vi "20210716_Scan with scanning mirror_center point_ver4.0.vi"(8 "Y Scan range (V)":dbl=0.2 min=-200.0 max=300.0, 9 "X Scan range (V)":dbl=0.2 min=-200.0 max=300.0, 10 "Y center (V)":dbl min=-200.0 max=300.0, 11 "X center (V)":dbl min=-200.0 max=300.0) -> ()   [LabVIEW 2015]
uses:
  Libraries/SR400/Public/Typedefs/Counter.ctl
  <vilib>/Analysis/1siggen.llb/Ramp Pattern by Samples.vi
  <vilib>/Analysis/NI_AALBase.lvlib
  Libraries/SR400/SR400.lvlib
panel:
  in  "file path":path
  out "SR400 counts":dbl
  in  "STOP\nSCAN":bool
  in  "Position from":enum16{"Left", "Right", "Control"}(ring)
  in  "Scan select":enum16{"Left", "Right"}(ring)
  in  "Position select":enum16{"Left", "Right", "Zero", "Control"}(ring)
  out "Current Y position (V)":dbl format="%#_4g"
  out "Current X position (V)":dbl format="%#_4g"
  out "Cursor_Y (V) 2":dbl format="%#.5f"
  out "Cursor_X (V) 2":dbl format="%#.5f"
  out "Cursor_Y position 2":i32
  out "Cursor_X position 2":i32
  out "X_Array 2":dbl[](array[numeric])
  out "Y_Array 2":dbl[](array[numeric])
  out "Rescanned Intensity Graph":dbl[][](graph)
  out "Count plot":dbl(graph)=137.0
  in  "stop monitoring":bool
  in  "Log":bool
  out "X_Array":dbl[](array[numeric])
  out "Y_Array":dbl[](array[numeric])
  in  "Scan":bool
  out "Cursor_Y (V)":dbl format="%#.5f"
  out "Cursor_X (V)":dbl format="%#.5f"
  in  "Go":bool
  in  "Stop program":bool
  out "Cursor_Y position":i32
  out "Cursor_X position":i32
  in  "Count Time Set":dbl[unit]=0.01
  in  "# of average":i32=1
  in  "VISA resource name":refnum<visa-resource-name>="GPIB0::18::INSTR"
  in  "Dwell time (ms)":i32=2
  out "Counts":dbl
  in  "Time delay bet. movement\n& measurement (ms)":i32=1
  in  "X data number(Ao1)":i32=150
  out "Max Value":dbl format="%#.2p"
  out "Max Y (V)":dbl format="%#.5f"
  out "Max X (V)":dbl format="%#.5f"
  out "Intensity Graph":dbl[][](graph)
  out "ao1_V":dbl
  out "ao1_index":i32
  out "ao0_V":dbl
  out "ao0_index":i32
  in  "Y data number(Ao0)":i32=150
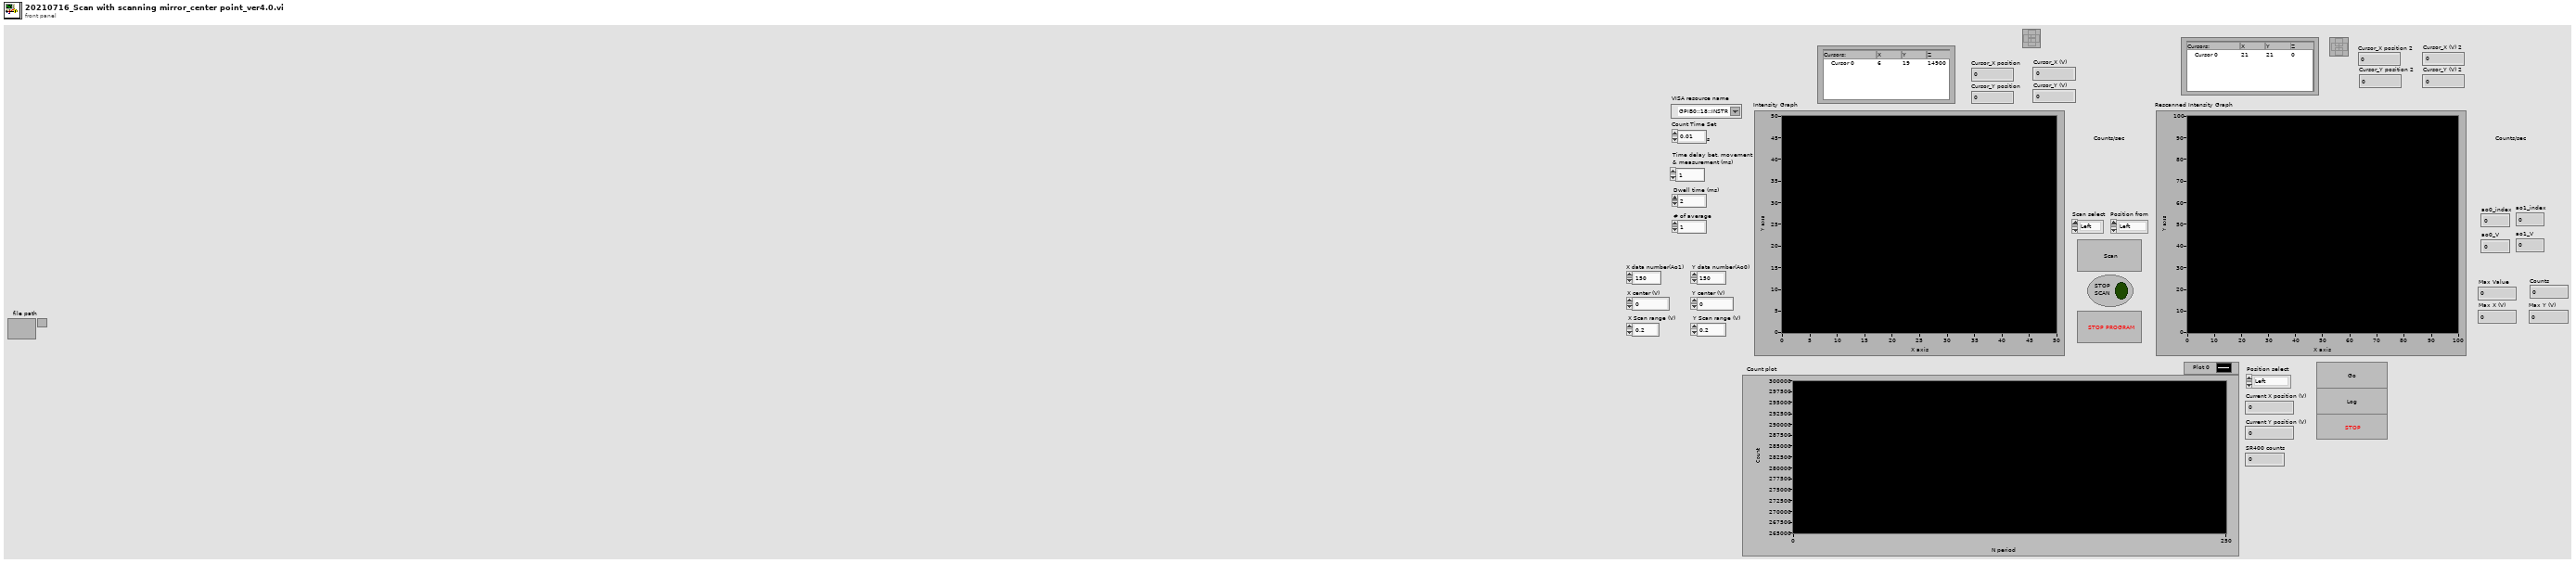
[diagram p1: front panel]
types:
  T1 = enum16{"open", "open or create", "create or replace", "create", "open (read only)"}
  T2 = typedef "SR400.lvlib/Counter.ctl" = enum16{"Counter A", "Counter B", "Counter T"}
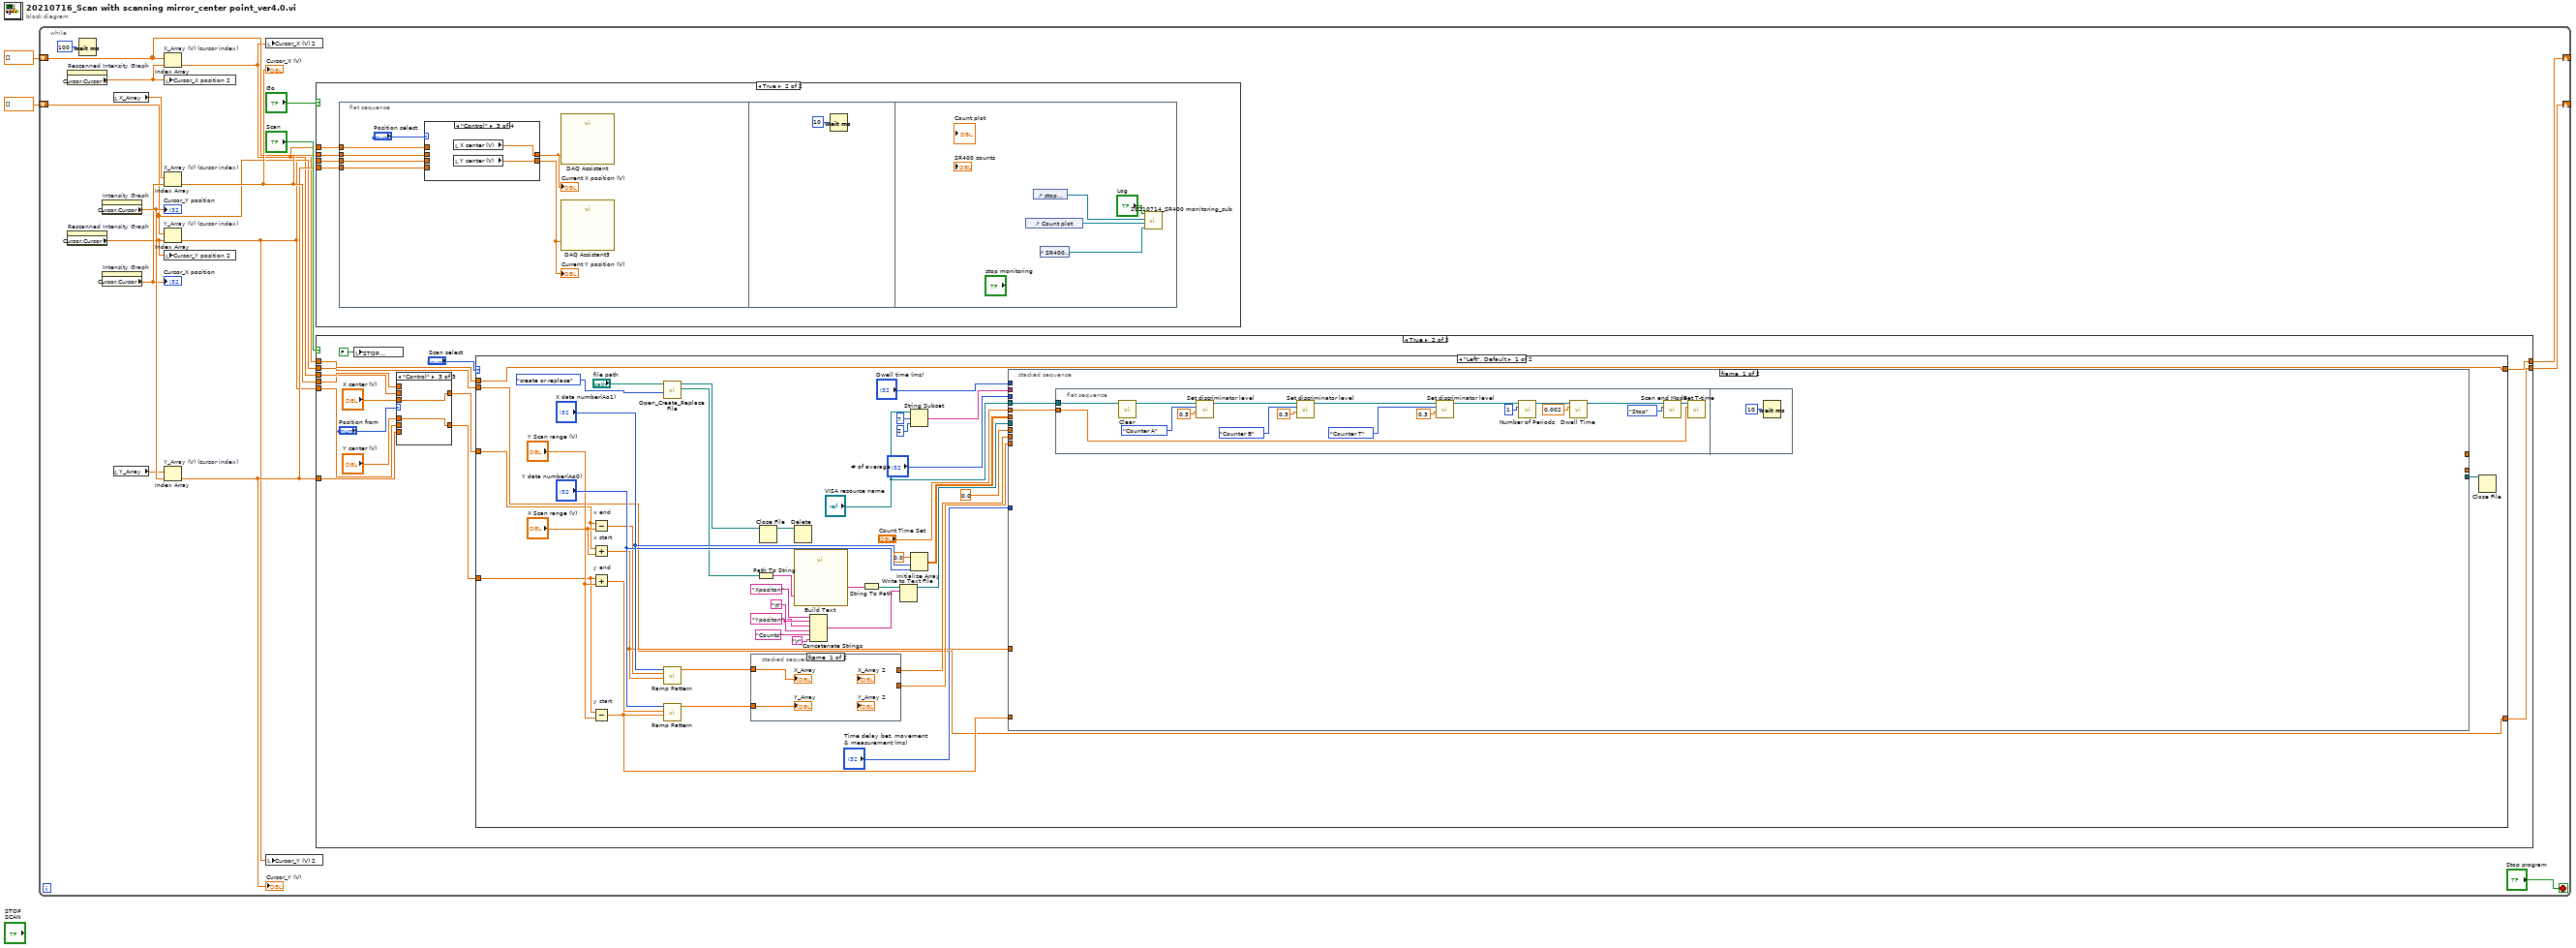
[diagram p0: block diagram]
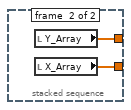
[diagram p5: hidden frame]
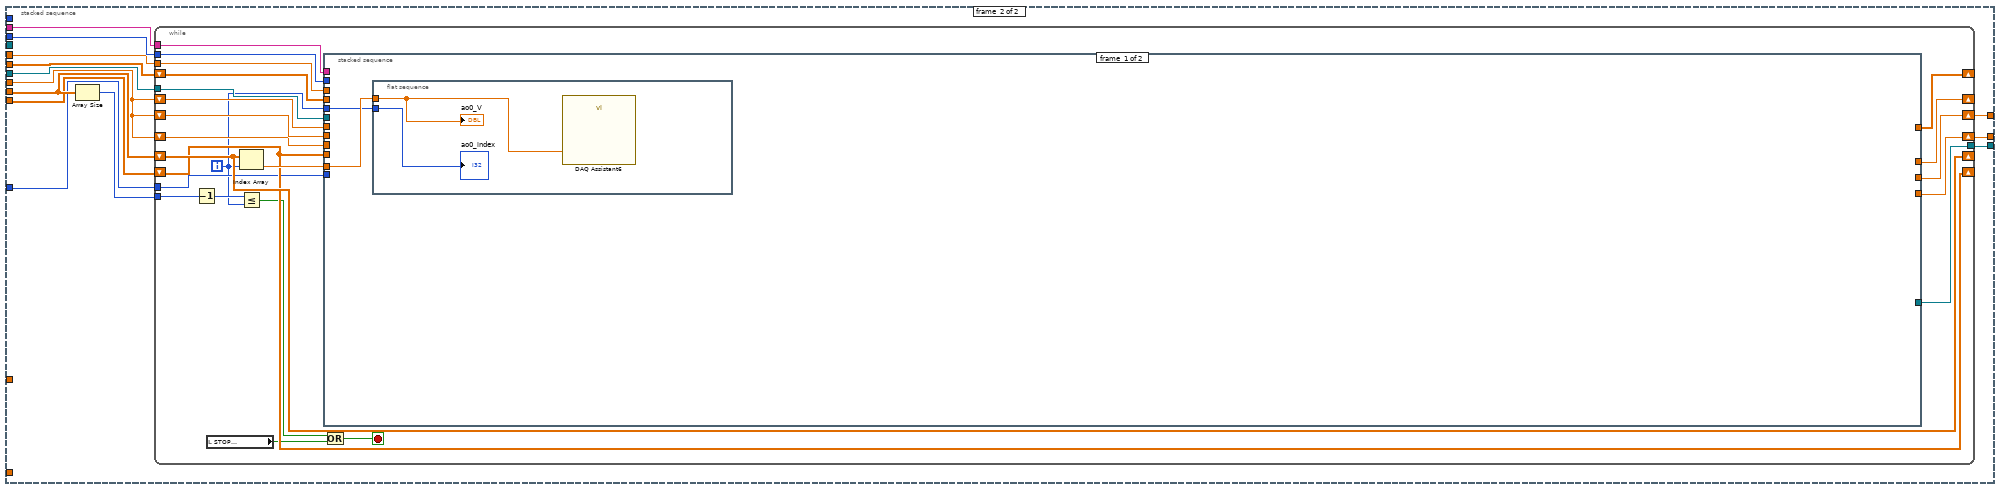
[diagram p6: hidden frame]
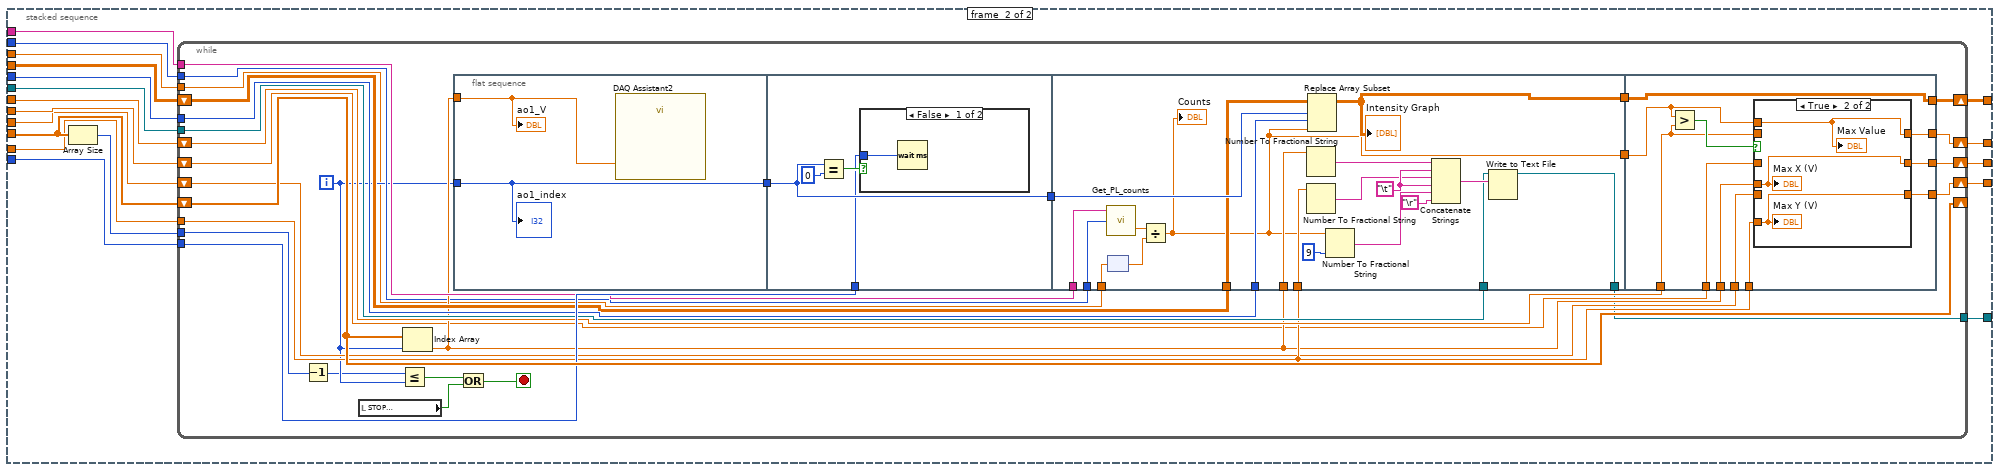
[diagram p7: hidden frame]
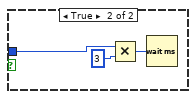
[diagram p8: hidden frame]
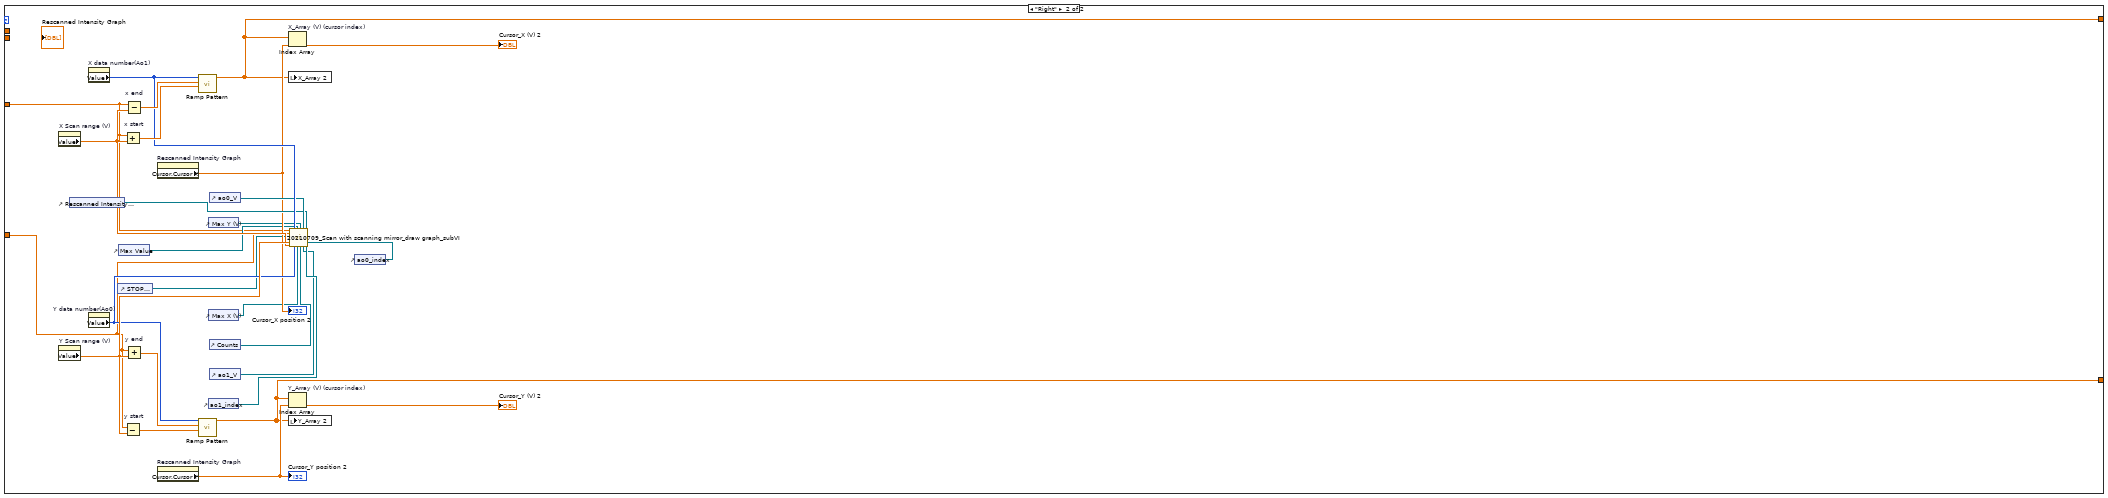
[diagram p10: hidden frame]
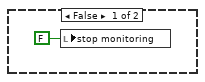
[diagram p11: hidden frame]
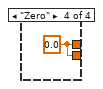
[diagram p14: hidden frame]
diagram:
  n1 = while {
    shift-right: [w10] -> _
    shift-left: dbl[] [] ("Ramp Pattern") -> [w6]
    shift-right: [w7] -> _
    shift-left: dbl[] [] ("Ramp Pattern") -> [w5]
    stop <- "Stop program" stop-if-true
    n2 = property on="Rescanned Intensity Graph" class="IntGraph (strict)"() -> ("Cursor.Cursor X"=w9:dbl)  [unwired: 2 in, 2 out]
    n3 = property on="Rescanned Intensity Graph" class="IntGraph (strict)"() -> ("Cursor.Cursor Y"=w8:dbl)  [unwired: 2 in, 2 out]
    n4 = Wait (ms)(milliseconds to wait=u32 100) -> ()  [unwired: 1 out]
    n5 = property on="Intensity Graph" class="IntGraph (strict)"() -> ("Cursor.Cursor Y"=w17:dbl)  [unwired: 2 in, 2 out]
    "Cursor_Y position" <- w17
    n6 = property on="Intensity Graph" class="IntGraph (strict)"() -> ("Cursor.Cursor X"=w16:dbl)  [unwired: 2 in, 2 out]
    "Cursor_X position" <- w16
    n7 = local read "X_Array"() -> (w15:dbl[])
    n8 = local read "Y_Array"() -> (w14:dbl[])
    n9 = Index Array "X_Array (V) (cursor index)"(array=w6, index=w9) -> (element=w4:dbl)
    n10 = local write "Cursor_X position 2"(w9) -> ()
    n11 = Index Array "X_Array (V) (cursor index)"(array=w15, index=w16) -> (element=w12:dbl)
    "Cursor_X (V)" <- w12
    n12 = Index Array "Y_Array (V) (cursor index)"(array=w5, index=w8) -> (element=w3:dbl)
    n13 = local write "Cursor_Y position 2"(w8) -> ()
    n14 = Index Array "Y_Array (V) (cursor index)"(array=w14, index=w17) -> (element=w11:dbl)
    "Cursor_Y (V)" <- w11
    n15 = local write "Cursor_X (V) 2"(w4) -> ()
    n16 = local write "Cursor_Y (V) 2"(w3) -> ()
    n17 = case shown="True" "Go" {
      tunnel: w12 -> [_ w276]
      tunnel: w11 -> [_ w275]
      tunnel: w4 -> [_ w274]
      tunnel: w3 -> [_ w273]
      frame False {
        n18 = local write "stop monitoring"(FALSE ("monitoring stop")) -> ()
      }
      frame True {
        n19 = flat-sequence {
          tunnel: w276 -> [w282]
          tunnel: w275 -> [w281]
          tunnel: w274 -> [w280]
          tunnel: w273 -> [w279]
          frame #0 {
            n20 = case shown="\"Control\"" "Position select" {
              tunnel: w282 -> [w285 _ _ _]
              tunnel: w281 -> [w284 _ _ _]
              tunnel: w280 -> [_ w287 _ _]
              tunnel: w279 -> [_ w286 _ _]
              tunnel: [w285 w287 w288 w290] -> w278
              tunnel: [w284 w286 w289 w290] -> w277
              frame "Left", Default {
              }
              frame "Right" {
              }
              frame "Control" {
                n21 = local read "X center (V)"() -> (w288:dbl)
                n22 = local read "Y center (V)"() -> (w289:dbl)
              }
              frame "Zero" {
                w290 = 0.0
              }
            }
            "Current X position (V)" <- w278
            "Current Y position (V)" <- w277
            n23 = call "DAQ Assistant"("data"=w278) -> ()  [unwired: 17 in, 2 out]
            n24 = call "DAQ Assistant3"("data"=w277) -> ()  [unwired: 17 in, 2 out]
          }
          frame #1 {
            n25 = Wait (ms)(milliseconds to wait=u32 10) -> ()  [unwired: 1 out]
          }
          frame #2 {
            n26 = control-ref of="Count plot"() -> (w295:refnum<vi>)
            n27 = control-ref of="stop monitoring"() -> (w294:refnum<vi>)
            n28 = control-ref of="SR400 counts"() -> (w292:refnum<vi>)
            n29 = call "20210714_SR400 monitoring_sub.vi"("DigNum Refnum"=w292, "Ctl Refnum"=w295, "stop Refnum"=w294, 11:"Log") -> ()  [unwired: 8 in]
          }
        }
      }
    }
    n30 = case shown="True" "Scan" {
      tunnel: w11 -> [_ w28]
      tunnel: w12 -> [_ w30]
      tunnel: [w22 w37] -> w10
      tunnel: [w21 w36] -> w7
      tunnel: w6 -> [w22 w34]
      tunnel: w5 -> [w21 w33]
      tunnel: w4 -> [_ w31]
      tunnel: w3 -> [_ w29]
      frame False {
      }
      frame True {
        n31 = local write "STOP\nSCAN"(FALSE ("STOP SCAN")) -> ()
        n32 = case shown="\"Control\"" "Position from" {
          tunnel: [w39 w41 w43] -> w27
          tunnel: w30 -> [w39 _ _]
          tunnel: w28 -> [w38 _ _]
          tunnel: [w38 w40 w42] -> w26
          tunnel: w31 -> [_ w41 _]
          tunnel: w29 -> [_ w40 _]
          tunnel: "X center (V)" -> [_ _ w43]
          tunnel: "Y center (V)" -> [_ _ w42]
          frame "Left", Default {
          }
          frame "Right" {
          }
          frame "Control" {
          }
        }
        n33 = case shown="\"Left\", Default" "Scan select" {
          tunnel: [w59 w252] -> w37
          tunnel: [w58 w251] -> w36
          tunnel: w34 -> [w59 _]
          tunnel: w33 -> [w58 _]
          tunnel: w27 -> [w53 w248]
          tunnel: w26 -> [w52 w247]
          frame "Left", Default {
            w65 = "\t"
            n34 = Subtract "x end"(x=w53, y="X Scan range (V)") -> (x-y=w72:dbl)
            n35 = Add "x start"(x=w53, y="X Scan range (V)") -> (x+y=w73:dbl)
            n36 = Add "y end"(x=w52, y="Y Scan range (V)") -> (x+y=w71:dbl)
            n37 = Subtract "y start"(x=w52, y="Y Scan range (V)") -> (x-y=w70:dbl)
            n38 = call <vilib>:"Open_Create_Replace File.vi"("function (open:0)"=T1."create or replace", "file path"="file path") -> ("new file path"=w50:path, "refnum"=w46:refnum<file>)  [unwired: 6 in, 2 out]
            n39 = call-poly <vilib>:"Ramp Pattern.vi"("start"=w73, "end"=w72, "samples"="X data number(Ao1)") -> ("Ramp Pattern"=w86:dbl[])  [unwired: 7 in, 1 out]
            n40 = call-poly <vilib>:"Ramp Pattern.vi"("start"=w70, "end"=w71, "samples"="Y data number(Ao0)") -> ("Ramp Pattern"=w85:dbl[])  [unwired: 7 in, 1 out]
            n41 = stacked-sequence {
              tunnel: [_ w90] -> w83
              tunnel: [_ w89] -> w84
              tunnel: w85 -> [w88 _]
              tunnel: w86 -> [w87 _]
              frame #0 {
                "Y_Array" <- w88
                "X_Array" <- w87
              }
              frame #1 {
                n42 = local read "Y_Array"() -> (w90:dbl[])
                n43 = local read "X_Array"() -> (w89:dbl[])
              }
            }
            n44 = Path To String(path=w50) -> (string=w45:string)
            n45 = Close File(refnum=w46) -> (path=w47:path)  [unwired: 1 in, 1 out]
            n46 = Delete(path (use dialog)=w47) -> ()  [unwired: 4 in, 3 out]
            n47 = call "Build Text"("a"=w45) -> ("Result"=w51:string)  [unwired: 13 in, 1 out]
            n48 = Concatenate Strings("Xpositon" ("string"), w65, "Ypositon" ("string"), w65, "Counts" ("string"), "\r") -> (w62:string)
            n49 = String To Path(string=w51) -> (path=w44:path)
            n50 = Write to Text File(file (use dialog)=w44, text=w62) -> (refnum out=w68:refnum<file>)  [unwired: 2 in, 2 out]
            n51 = String Subset(string="VISA resource name", offset (0)=7, length (rest)=2 ("length (rest)")) -> (substring=w55:string)
            n52 = Initialize Array(0.0, "X data number(Ao1)", "Y data number(Ao0)") -> (w78:dbl[][])
            n53 = stacked-sequence {
              tunnel: w83 -> [_ w124]
              tunnel: w84 -> [_ w123]
              tunnel: "Time delay bet. movement\n& measurement (ms)" -> [_ w122]
              tunnel: w55 -> [_ w121]
              tunnel: w78 -> [_ w120]
              tunnel: w68 -> [_ w119]
              tunnel: [_ w118] -> w69
              tunnel: w73 -> [_ _]
              tunnel: w70 -> [_ _]
              tunnel: 0.0 -> [_ w117]
              tunnel: "Dwell time (ms)" -> [_ _]
              tunnel: [_ w116] -> _
              tunnel: [_ w115] -> _
              tunnel: "# of average" -> [_ w114]
              tunnel: "Count Time Set" -> [w92 w112]
              tunnel: "VISA resource name" -> [w91 _]
              frame #0 {
                n54 = flat-sequence {
                  tunnel: w92 -> [w94]
                  tunnel: w91 -> [w93]
                  frame #0 {
                    n55 = call "Clear.vi"("VISA resource name"=w93) -> ("VISA resource name out"=w110:refnum<visa-resource-name>)  [unwired: 9 in, 1 out]
                    n56 = call "Set discriminator level.vi"("Level (-0.034 V)"=0.3, "Discriminator (def: A)"=Counter."Counter A", "VISA resource name"=w110) -> ("VISA resource name out"=w107:refnum<visa-resource-name>)  [unwired: 7 in, 1 out]
                    n57 = call "Set discriminator level.vi"("Level (-0.034 V)"=0.3, "Discriminator (def: A)"=Counter."Counter B", "VISA resource name"=w107) -> ("VISA resource name out"=w104:refnum<visa-resource-name>)  [unwired: 7 in, 1 out]
                    n58 = call "Set discriminator level.vi"("Level (-0.034 V)"=0.3, "Discriminator (def: A)"=Counter."Counter T", "VISA resource name"=w104) -> ("VISA resource name out"=w101:refnum<visa-resource-name>)  [unwired: 7 in, 1 out]
                    n59 = call "Number of Periods.vi"("# of periods (def: 1)"=1, "VISA resource name"=w101) -> ("VISA resource name out"=w99:refnum<visa-resource-name>)  [unwired: 8 in, 1 out]
                    n60 = call "Dwell Time.vi"("Dwell time (0.002 s)"=0.002, "VISA resource name"=w99) -> ("VISA resource name out"=w97:refnum<visa-resource-name>)  [unwired: 8 in, 1 out]
                    n61 = call "Scan end Mode.vi"("Scan End Mode (Def: Stop)"=enum16{"Stop", "Start"}."Stop", "VISA resource name"=w97) -> ("VISA resource name out"=w95:refnum<visa-resource-name>)  [unwired: 8 in, 1 out]
                    n62 = call "Set T-time.vi"("Count Time Set"=w94, "VISA resource name"=w95) -> ()  [unwired: 5 in, 3 out]
                  }
                  frame #1 {
                    n63 = Wait (ms)(milliseconds to wait=u32 10) -> ()  [unwired: 1 out]
                  }
                }
              }
              frame #1 {
                n64 = Array Size(array=w124) -> (size(s)=w113:i32)
                n65 = while {
                  shift-right: [w146] -> _
                  shift-left: w124 -> [w146]
                  shift-right: [w145] -> _
                  shift-left: w123 -> [w145]
                  tunnel: w122 -> [w144]
                  tunnel: w121 -> [w143]
                  shift-right: [w140] -> _
                  shift-left: w120 -> [w142]
                  tunnel: w119 -> [w141]
                  tunnel: [w139] -> w118
                  shift-right: [w138] -> w115
                  shift-left: w117 -> [w133]
                  shift-right: [w136] -> _
                  shift-left: w117 -> [w134]
                  shift-right: [w137] -> w116
                  shift-left: w117 -> [w135]
                  tunnel: w114 -> [w132]
                  tunnel: w113 -> [w128]
                  tunnel: w112 -> [w125]
                  i -> [w127]
                  stop <- w126 stop-if-true
                  n66 = Decrement(x=w128) -> (x-1=w129:i32)
                  n67 = local read "STOP\nSCAN"() -> (w131:bool)
                  n68 = Index Array(array=w146, index=w127) -> (element=w147:dbl)
                  n69 = Less Or Equal?(x=w129, y=w127) -> (x <= y?=w130:bool)
                  n70 = stacked-sequence {
                    tunnel: w147 -> [w149 w164]
                    tunnel: w145 -> [_ w169]
                    tunnel: w144 -> [_ w168]
                    tunnel: w127 -> [w148 w166]
                    tunnel: w143 -> [_ w167]
                    tunnel: w142 -> [_ w165]
                    tunnel: w141 -> [_ w163]
                    tunnel: [_ w162] -> w140
                    tunnel: [_ w161] -> w139
                    tunnel: [_ w160] -> w138
                    tunnel: [_ w159] -> w137
                    tunnel: [_ w158] -> w136
                    tunnel: w135 -> [_ w157]
                    tunnel: w134 -> [_ w156]
                    tunnel: w133 -> [_ w155]
                    tunnel: w132 -> [_ w154]
                    tunnel: w125 -> [_ w152]
                    frame #0 {
                      n71 = flat-sequence {
                        tunnel: w149 -> [w150]
                        tunnel: w148 -> [w151]
                        frame #0 {
                          n72 = call "DAQ Assistant6"("data"=w150) -> ()  [unwired: 17 in, 2 out]
                          "ao0_V" <- w150
                          "ao0_index" <- w151
                        }
                      }
                    }
                    frame #1 {
                      n73 = Array Size(array=w169) -> (size(s)=w153:i32)
                      n74 = while {
                        shift-right: [w197] -> _
                        shift-left: w169 -> [w197]
                        tunnel: w168 -> [w196]
                        tunnel: w167 -> [w195]
                        tunnel: w166 -> [w193]
                        shift-right: [w191] -> w162
                        shift-left: w165 -> [w192]
                        tunnel: w164 -> [w185]
                        tunnel: w163 -> [w190]
                        shift-right: [w187] -> w158
                        shift-left: w156 -> [w186]
                        shift-right: [w183] -> w160
                        shift-left: w155 -> [w181]
                        shift-right: [w182] -> w159
                        shift-left: w157 -> [w180]
                        tunnel: [w179] -> w161
                        tunnel: w154 -> [w177]
                        tunnel: w153 -> [w174]
                        tunnel: w152 -> [w170]
                        i -> [w176]
                        stop <- w171 stop-if-true
                        n75 = Decrement(x=w174) -> (x-1=w175:i32)
                        n76 = local read "STOP\nSCAN"() -> (w172:bool)
                        n77 = Less Or Equal?(x=w175, y=w176) -> (x <= y?=w173:bool)
                        n78 = Index Array(array=w197, index=w176) -> (element=w184:dbl)
                        n79 = flat-sequence {
                          tunnel: w184 -> [w199]
                          tunnel: w176 -> [w198]
                          tunnel: [w198] -> w178
                          tunnel: w196 -> [w200]
                          tunnel: [w202] -> w194
                          tunnel: w178 -> [w202]
                          tunnel: w195 -> [w213]
                          tunnel: w194 -> [w228]
                          tunnel: w193 -> [w227]
                          tunnel: w192 -> [w226]
                          tunnel: w184 -> [w218]
                          tunnel: w185 -> [w217]
                          tunnel: w190 -> [w215]
                          tunnel: [w225] -> w189
                          tunnel: [w211] -> w188
                          tunnel: [w214] -> w179
                          tunnel: w177 -> [w212]
                          tunnel: w170 -> [w208]
                          tunnel: [w239] -> w191
                          tunnel: w189 -> [w239]
                          tunnel: w188 -> [w229]
                          tunnel: [w237] -> w187
                          tunnel: w186 -> [w230]
                          tunnel: w185 -> [w236]
                          tunnel: w184 -> [w235]
                          tunnel: [w234] -> w183
                          tunnel: [w233] -> w182
                          tunnel: w181 -> [w232]
                          tunnel: w180 -> [w231]
                          frame #0 {
                            n80 = call "DAQ Assistant2"("data"=w199) -> ()  [unwired: 17 in, 2 out]
                            "ao1_V" <- w199
                            "ao1_index" <- w198
                          }
                          frame #1 {
                            n81 = Equal?(x=w202, y=0) -> (x = y?=w203:bool)
                            n82 = case shown="False" w203 {
                              tunnel: w200 -> [w204 w206]
                              frame False {
                                n83 = Wait (ms)(milliseconds to wait=w204) -> ()  [unwired: 1 out]
                              }
                              frame True {
                                n84 = Multiply(x=w206, y=3) -> (x*y=w207:i32)
                                n85 = Wait (ms)(milliseconds to wait=w207) -> ()  [unwired: 1 out]
                              }
                            }
                          }
                          frame #2 {
                            w224 = "\t"
                            n86 = call "Get_PL_counts.vi"("# of average"=w212, "SR400 GPIB Address"=w213) -> ("Averaged counts"=w210:dbl)  [unwired: 2 in]
                            n87 = node(w208) -> (w209:dbl)
                            n88 = Divide(x=w210, y=w209) -> (x/y=w211:dbl)
                            "Counts" <- w211
                            n89 = Number To Fractional String(number=w218) -> (F-format string=w219:string)  [unwired: 3 in]
                            n90 = Number To Fractional String(number=w217) -> (F-format string=w216:string)  [unwired: 3 in]
                            n91 = Replace Array Subset(array=w226, new element=w211, index (row)=w228, index (col)=w227) -> (w225:dbl[][])
                            "Intensity Graph" <- w225
                            n92 = Number To Fractional String(number=w211, precision (6)=i16 9) -> (F-format string=w220:string)  [unwired: 2 in]
                            n93 = Concatenate Strings(w219, w224, w216, w224, w220, "\r") -> (w222:string)
                            n94 = Write to Text File(file (use dialog)=w215, text=w222) -> (refnum out=w214:refnum<file>)  [unwired: 2 in, 2 out]
                          }
                          frame #3 {
                            n95 = Greater?(x=w229, y=w230) -> (0:w238:bool)
                            n96 = case shown="True" w238 {
                              tunnel: w229 -> [_ w245]
                              tunnel: [w242 w245] -> w237
                              tunnel: w230 -> [w242 _]
                              tunnel: w236 -> [_ w244]
                              tunnel: w235 -> [_ w243]
                              tunnel: [w241 w244] -> w234
                              tunnel: [w240 w243] -> w233
                              tunnel: w232 -> [w241 _]
                              tunnel: w231 -> [w240 _]
                              frame False {
                              }
                              frame True {
                                "Max Value" <- w245
                                "Max Y (V)" <- w244
                                "Max X (V)" <- w243
                              }
                            }
                          }
                        }
                        n97 = Or(x=w173, y=w172) -> (x .or. y?=w171:bool)
                      }
                    }
                  }
                  n98 = Or(x=w130, y=w131) -> (x .or. y?=w126:bool)
                }
              }
            }
            n99 = Close File(refnum=w69) -> ()  [unwired: 1 in, 2 out]
          }
          frame "Right" {
            n100 = property on="X Scan range (V)" class="DigNum (strict)"() -> ("Value"=w267:dbl)  [unwired: 2 in, 2 out]
            n101 = property on="Y Scan range (V)" class="DigNum (strict)"() -> ("Value"=w271:dbl)  [unwired: 2 in, 2 out]
            n102 = control-ref of="Rescanned Intensity Graph"() -> (w259:refnum<vi>)
            n103 = property on="X data number(Ao1)" class="DigNum (strict)"() -> ("Value"=w264:i32)  [unwired: 2 in, 2 out]
            n104 = property on="Y data number(Ao0)" class="DigNum (strict)"() -> ("Value"=w268:i32)  [unwired: 2 in, 2 out]
            n105 = control-ref of="STOP\nSCAN"() -> (w246:refnum<vi>)
            n106 = control-ref of="Max Value"() -> (w250:refnum<vi>)
            n107 = Add "x start"(x=w248, y=w267) -> (x+y=w265:dbl)
            n108 = Subtract "y start"(x=w247, y=w271) -> (x-y=w269:dbl)
            n109 = Subtract "x end"(x=w248, y=w267) -> (x-y=w266:dbl)
            n110 = Add "y end"(x=w247, y=w271) -> (x+y=w270:dbl)
            n111 = property on="Rescanned Intensity Graph" class="IntGraph (strict)"() -> ("Cursor.Cursor X"=w258:dbl)  [unwired: 2 in, 2 out]
            "Cursor_X position 2" <- w258
            n112 = property on="Rescanned Intensity Graph" class="IntGraph (strict)"() -> ("Cursor.Cursor Y"=w257:dbl)  [unwired: 2 in, 2 out]
            "Cursor_Y position 2" <- w257
            n113 = call-poly <vilib>:"Ramp Pattern.vi"("start"=w265, "end"=w266, "samples"=w264) -> ("Ramp Pattern"=w252:dbl[])  [unwired: 7 in, 1 out]
            n114 = call-poly <vilib>:"Ramp Pattern.vi"("start"=w269, "end"=w270, "samples"=w268) -> ("Ramp Pattern"=w251:dbl[])  [unwired: 7 in, 1 out]
            n115 = control-ref of="Max Y (V)"() -> (w253:refnum<vi>)
            n116 = control-ref of="Max X (V)"() -> (w254:refnum<vi>)
            n117 = control-ref of="ao1_index"() -> (w263:refnum<vi>)
            n118 = control-ref of="ao0_V"() -> (w261:refnum<vi>)
            n119 = control-ref of="Counts"() -> (w249:refnum<vi>)
            n120 = control-ref of="ao1_V"() -> (w260:refnum<vi>)
            n121 = Index Array "X_Array (V) (cursor index)"(array=w252, index=w258) -> (element=→"Cursor_X (V) 2":dbl)
            n122 = local write "X_Array 2"(w252) -> ()
            n123 = Index Array "Y_Array (V) (cursor index)"(array=w251, index=w257) -> (element=→"Cursor_Y (V) 2":dbl)
            n124 = local write "Y_Array 2"(w251) -> ()
            n125 = control-ref of="ao0_index"() -> (w262:refnum<vi>)
            n126 = call "20210709_Scan with scanning mirror_draw graph_subVI.vi"("X center (V)"=w248, "Y center (V)"=w247, "Bool Refnum"=w246, "X Scan range (V)"=w271, "Y Scan range (V)"=w267, "X data number(Ao1)"=w264, "Y data number(Ao0)"=w268, "DigNum Refnum 7"=w250, "DigNum Refnum 4"=w254, "DigNum Refnum 3"=w253, "DigNum Refnum 8"=w249, "DigNum Refnum 5"=w261, "DigNum Refnum 6"=w260, "IntGraph Refnum"=w259, "DigNum Refnum"=w262, "DigNum Refnum 2"=w263) -> ()  [unwired: 3 in, 1 out]
          }
        }
      }
    }
  }
